vi "Quick Usb Flush RS232.vi"(8 "error in (no error)":errorcluster, 10 "portNum":u8, 11 "hDevice":u32) -> (0 "error out":errorcluster, 2 "function return":i32, 3 "hDevice out":u32)   [LabVIEW 2011, in "QuickUSB.lvlib"]
doc: "QUSBLIB QRETURN QuickUsbFlushRS232(\n QHANDLE hDevice, \n QBYTE portNum\n);"
uses:
  QuickUSB.lvlib
  QuickUSB.dll
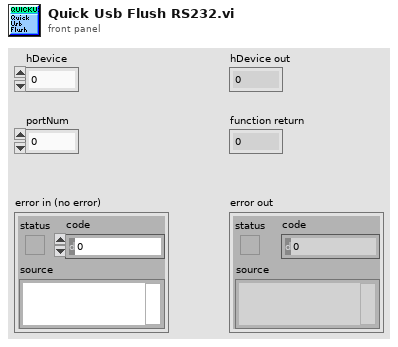
[diagram p1: front panel]
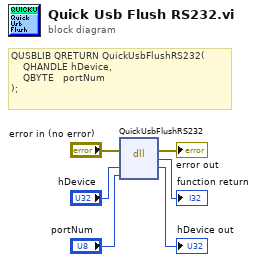
[diagram p0: block diagram]
diagram:
  # "QUSBLIB QRETURN QuickUsbFlushRS232(\n    QHANDLE hDevice, \n    QBYTE   portNum\n);"
  n1 = dll-call lib="C:/QuickUSB/QuickUSB.*" fn="QuickUsbFlushRS232"(error in="error in (no error)", "hDevice"="hDevice", "portNum"="portNum") -> (error out=→"error out":errorcluster, →"function return":i32, "hDevice"=→"hDevice out":u32)  [unwired: 3 in, 1 out]
